vi "LJU3_V2T.vi"(11 "voltage_array":dbl[](array[numeric])) -> (0 "V_loop_mean":dbl format="%.6f", 1 "array_T_F":dbl[](array[numeric]), 4 "External CJC (F)":dbl, 6 "Internal CJC (F)":dbl)   [LabVIEW 2019]
uses:
  <vilib>/Analysis/baseanly.llb/Mean (DBL).vi
  <vilib>/Analysis/NI_AALBase.lvlib
panel:
  out "array_T_K":dbl[](array[numeric])
  out "array_T_C":dbl[](array[numeric])
  out "External CJC (V)":dbl
  out "loop_voltages":dbl[](array[numeric])
  out "Internal CJC (K)":dbl
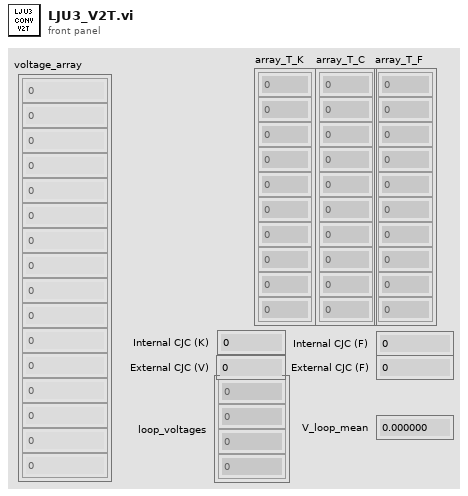
[diagram p1: front panel]
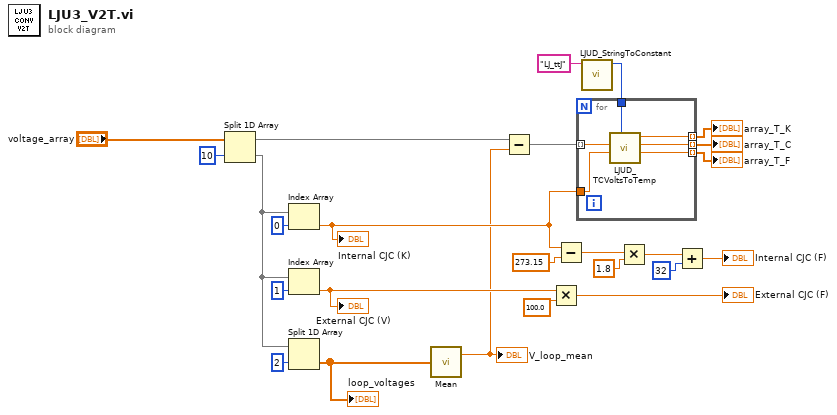
[diagram p0: block diagram]
diagram:
  n1 = Split 1D Array(array="voltage_array", index=10) -> (first subarray=w15:dbl[], second subarray=w10:dbl[])
  n2 = Index Array(array=w10, index=0) -> (element=w6:dbl)
  "Internal CJC (K)" <- w6
  n3 = Index Array(array=w10, index=1) -> (element=w5:dbl)
  "External CJC (V)" <- w5
  n4 = Split 1D Array(array=w10, index=2) -> (second subarray=w7:dbl[])  [unwired: 1 out]
  "loop_voltages" <- w7
  n5 = call-poly <vilib>:"Mean.vi"("X"=w7) -> ("mean"=w3:dbl)  [unwired: 1 out]
  "V_loop_mean" <- w3
  n6 = Subtract(x=w15, y=w3) -> (x-y=w4:dbl[])
  n7 = Multiply(x=w5, y=100.0) -> (x*y=→"External CJC (F)":dbl)
  n8 = Subtract(x=w6, y=273.15) -> (x-y=w23:dbl)
  n9 = call "LJUD_StringToConstant.vi"("String"="LJ_ttJ") -> ("Constant Number"=w17:i32)  [unwired: 9 in, 1 out]
  n10 = for {
    tunnel: w4 -> [w31] mode=indexing
    tunnel: w17 -> [w30]
    tunnel: [w29] -> w16 mode=indexing
    tunnel: w6 -> [w28]
    tunnel: [w27] -> w1 mode=indexing
    tunnel: [w26] -> w2 mode=indexing
    n11 = call "LJUD_TCVoltsToTemp.vi"("TCType"=w30, "CJTempK"=w28, "TCVolts"=w31) -> ("TCTempF"=w29:dbl, "TCTempC"=w26:dbl, "TCTempK"=w27:dbl)  [unwired: 5 in, 1 out]
  }
  "array_T_F" <- w16
  "array_T_C" <- w2
  "array_T_K" <- w1
  n12 = Multiply(x=w23, y=1.8) -> (x*y=w21:dbl)
  n13 = Add(x=w21, y=32) -> (x+y=→"Internal CJC (F)":dbl)
